vi "Configure DM-RS Sequence Generation.vi"(4 "nSCID (0)":i32, 5 "DMRS ID (0)":i32, 6 "Initialization (Physical Cell ID Used)":i32(ring) items=["Physical Cell ID Used", "DMRS ID Used"], 7 "Allocation (1)":T1=1, 8 "error in (no error)":errorcluster, 9 "CC (1)":T2=1, 10 "Instance (1)":T3=1, 11 "VISA resource name":refnum<visa-resource-name>) -> (0 "error out":errorcluster, 3 "VISA resource name out":refnum<visa-resource-name>)   [LabVIEW 2020, in "Rohde&Schwarz CMWXP NR FR1 Measurement.lvlib"]
doc: "Configures the initialization of the DM-RS sequence generation, for carrier <no>, allocation <a>.\n\nAttribute:\nRSCMWXPNRFR1M_ATTR_DR_MS_SEQUENCE_GENERATION\n\nRemote-control command:\nCONFigure:NRSub:MEAS<i>[:CC<no>]:ALLocation<a>:PUSCh:SGENeration"
uses:
  <instrlib>/Rohde&Schwarz CMWXP NR FR1 Measurement/Rohde&Schwarz CMWXP NR FR1 Measurement.lvlib
  <instrlib>/Rohde&Schwarz CMWXP NR FR1 Measurement/Private/_Instance.ctl
  <instrlib>/Rohde&Schwarz CMWXP NR FR1 Measurement/Private/_Carrier Component.ctl
  <instrlib>/Rohde&Schwarz CMWXP NR FR1 Measurement/Private/_Allocation.ctl
  <instrlib>/Rohde&Schwarz CMWXP NR FR1 Measurement/Private/rsidr_core.llb/rsidr_core.lvlib
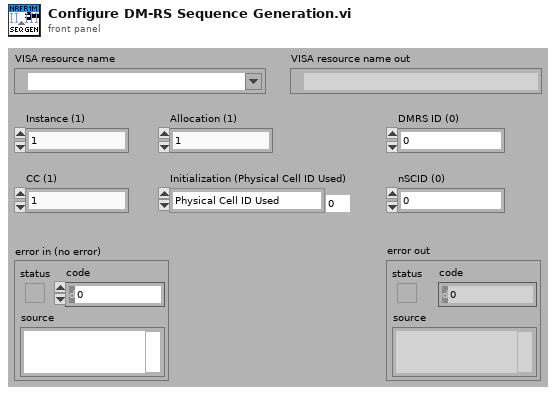
[diagram p1: front panel]
types:
  T1 = typedef "Rohde&Schwarz CMWXP NR FR1 Measurement.lvlib/_Allocation.ctl" = i32
  T2 = typedef "Rohde&Schwarz CMWXP NR FR1 Measurement.lvlib/_Carrier Component.ctl" = i32
  T3 = typedef "Rohde&Schwarz CMWXP NR FR1 Measurement.lvlib/_Instance.ctl" = i32
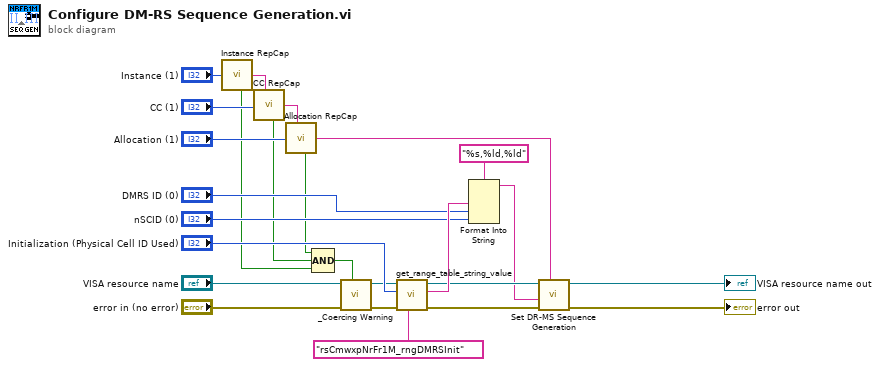
[diagram p0: block diagram]
diagram:
  n1 = call <instrlib>:"Instance RepCap.vi"("Instance In"="Instance (1)") -> ("In Range?"=w2:bool, "RepCap Identifier Out"=w22:string)  [unwired: 1 in]
  n2 = call <instrlib>:"CC RepCap.vi"("CC In"="CC (1)", "RepCap String In (\"\")"=w22) -> ("In Range?"=w3:bool, "RepCap Identifier Out"=w21:string)
  n3 = call <instrlib>:"Allocation RepCap.vi"("Allocation In"="Allocation (1)", "RepCap String In (\"\")"=w21) -> ("In Range?"=w1:bool, "RepCap Identifier Out"=w20:string)
  n4 = Compound Arithmetic op=AND(w1, w3, w2) -> (w4:bool)
  n5 = call <instrlib>:"_Coercing Warning.vi"("In Range?"=w4, "error in (no error)"="error in (no error)", "VISA resource name"="VISA resource name") -> ("error out"=w6:errorcluster, "VISA resource name out"=w5:refnum<visa-resource-name>)  [unwired: 7 in]
  n6 = call <instrlib>:"get_range_table_string_value.vi"("Range Table ID in"="rsCmwxpNrFr1M_rngDMRSInit", "error in"=w6, "I32 input"="Initialization (Physical Cell ID Used)", "VISA resource name"=w5) -> ("error out"=w13:errorcluster, "String Value out"=w16:string, "VISA resource name out"=w10:refnum<visa-resource-name>)  [unwired: 5 in]
  n7 = Format Into String(format string="%s,%ld,%ld", w16, "DMRS ID (0)", "nSCID (0)") -> (resulting string=w9:string)  [unwired: 2 in, 1 out]
  n8 = call "Set DR-MS Sequence Generation"("Repeated Capabilities"=w20, "error in (no error)"=w13, "DR-MS Sequence Generation ()"=w9, "instrument handle"=w10) -> ("error out"=→"error out":errorcluster, "instrument handle out"=→"VISA resource name out":refnum<visa-resource-name>)  [unwired: 6 in]
